vi "Username and Password.vi"() -> (1 "User name: 2":string, 2 "Logged In?":bool)   [LabVIEW 2012]
panel:
  in  "Cancel":bool
  in  "Password:":string
  in  "User name:":string
  in  "OK":bool
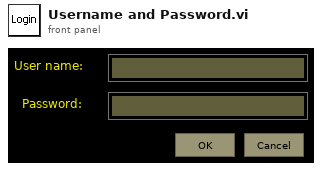
[diagram p1: front panel]
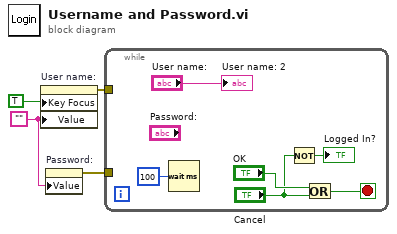
[diagram p0: block diagram]
diagram:
  w4 = ""
  n1 = property on="User name:" class="Str"("Key Focus"=TRUE, "Value"=w4) -> (error out=w3:errorcluster)  [unwired: 2 in, 1 out]
  n2 = property on="Password:" class="Str"("Value"=w4) -> (error out=w2:errorcluster)  [unwired: 2 in, 1 out]
  n3 = while {
    tunnel: w2 -> [_]
    tunnel: w3 -> [_]
    stop <- w9 stop-if-true
    n4 = Wait (ms)(milliseconds to wait=u32 100) -> ()  [unwired: 1 out]
    n5 = Not(x="Cancel") -> (.not. x?=→"Logged In?":bool)
    n6 = Or(x="OK", y="Cancel") -> (x .or. y?=w9:bool)
    "User name: 2" <- "User name:"
  }
